vi "Initialize.vi"(5 "Password":string, 7 "Username":string, 8 "error in (no error)":errorcluster, 10 "Address":string, 11 "FTP in":refnum<class "FTP.lvclass">) -> (0 "error out":errorcluster, 3 "FTP out":refnum<class "FTP.lvclass">)   [LabVIEW 2015, in "RT Management.lvlib" / "FTP.lvclass"]
uses:
  FTP.lvclass
  File Transfer Behavior/File Transfer Behavior.lvclass/File Transfer Behavior.ctl
  FTP.lvclass/FTP.ctl
  File Transfer Behavior/Set Address.vi
  File Transfer Behavior/Set Username.vi
  File Transfer Behavior/Set Password.vi
  File Transfer Behavior/Get Username.vi
  File Transfer Behavior/Get Password.vi
  File Transfer Behavior/Get Address.vi
  Set Session.vi
  <vilib>/FTP/NI_FTP.lvlib
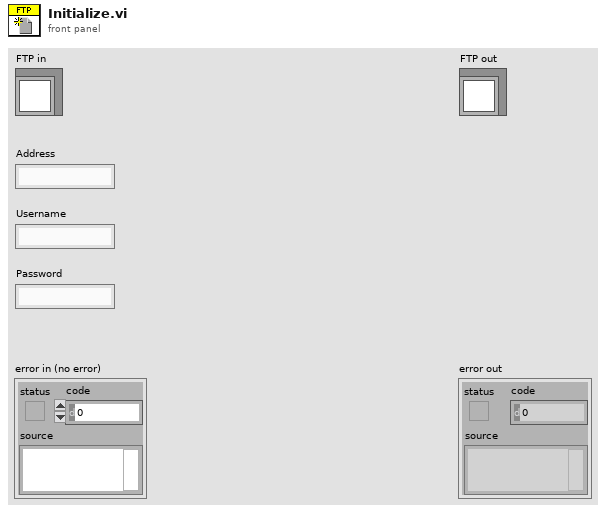
[diagram p1: front panel]
types:
  T1 = typedef "NI_FTP.lvlib/FTP Session.ctl" = refnum<k5>
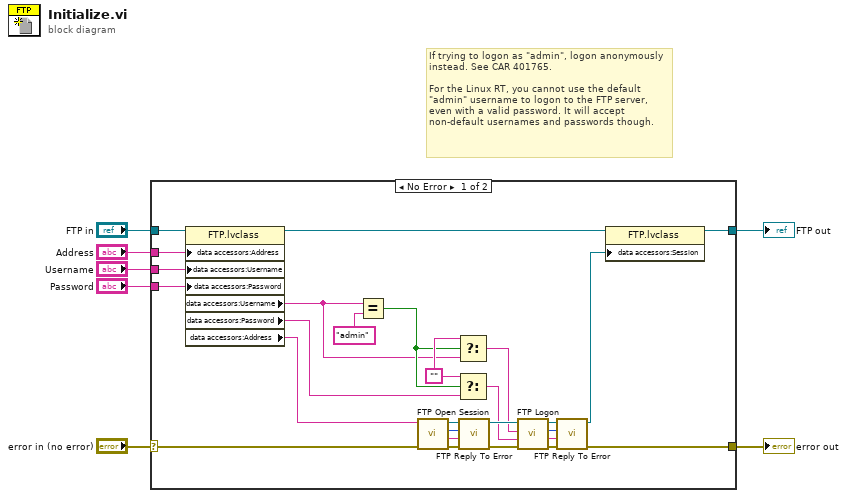
[diagram p0: block diagram]
diagram:
  # "If trying to logon as \"admin\", logon anonymously instead. See CAR 401765.\n\nFor the Linux RT, you cannot use the default \"admin\" username to logon to the FTP server, even with a valid password. It will accept non-default usernames and passwords though."
  n1 = case shown="No Error" "error in (no error)" {
    selector: "error in (no error)" -> [w21 w35]
    tunnel: [w29 w35] -> w7
    tunnel: "FTP in" -> [w15 w36]
    tunnel: [w22 w36] -> w6
    tunnel: "Address" -> [w13 _]
    tunnel: "Username" -> [w12 _]
    tunnel: "Password" -> [w11 _]
    frame No Error {
      w18 = ""
      n2 = property class="FTP.lvclass"(reference=w15, "data accessors:Address"=w13, "data accessors:Username"=w12, "data accessors:Password"=w11) -> (reference out=w14:refnum<class "FTP.lvclass">, "data accessors:Username"=w8:string, "data accessors:Password"=w9:string, "data accessors:Address"=w28:string)  [unwired: 1 in, 1 out]
      n3 = Equal?(x=w8, y="admin") -> (x = y?=w10:bool)
      n4 = call <vilib>:"FTP Open Session.vi"("error in (no error)"=w21, "address"=w28) -> ("error out"=w26:errorcluster, "reply string"=w25:string, "reply code"=w24:i32, "ftp session"=w27:T1)  [unwired: 6 in]
      n5 = Select(t=w18, s=w10, f=w8) -> (s? t:f=w16:string)
      n6 = Select(t=w18, s=w10, f=w9) -> (s? t:f=w17:string)
      n7 = call <vilib>:"FTP Reply To Error.vi"("error in (no error)"=w26, "reply string in"=w25, "reply code in"=w24, "ftp session"=w27) -> ("error out"=w23:errorcluster, "ftp session out"=w34:T1)  [unwired: 2 out]
      n8 = call <vilib>:"FTP Logon.vi"("error in (no error)"=w23, "password"=w17, "user"=w16, "ftp session"=w34) -> ("error out"=w33:errorcluster, "reply string"=w30:string, "reply code"=w31:i32, "ftp session out"=w32:T1)  [unwired: 4 in]
      n9 = call <vilib>:"FTP Reply To Error.vi"("error in (no error)"=w33, "reply string in"=w30, "reply code in"=w31, "ftp session"=w32) -> ("error out"=w29:errorcluster, "ftp session out"=w20:T1)  [unwired: 2 out]
      n10 = property class="FTP.lvclass"(reference=w14, "data accessors:Session"=w20) -> (reference out=w22:refnum<class "FTP.lvclass">)  [unwired: 1 in, 1 out]
    }
    frame Error {
    }
  }
  "error out" <- w7
  "FTP out" <- w6
